vi "Wait For Trigger.vi"(8 "error in":errorcluster, 10 "Cancel":bool, 11 "VISA resource name":refnum<visa-resource-name>) -> (0 "error out":errorcluster, 2 "Trigger Activated":bool, 3 "VISA resource name out":refnum<visa-resource-name>)   [LabVIEW 2020]
uses:
  <vilib>/Instr/_visa.llb/VISA Flush IO Buffer Mask.ctl
panel:
  out "read buffer":string
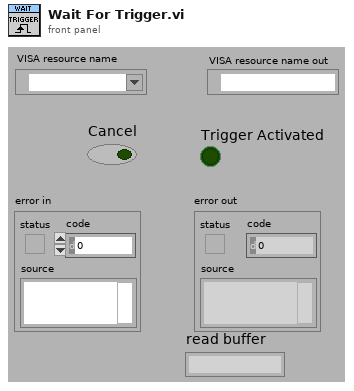
[diagram p1: front panel]
types:
  T1 = typedef "VISA Flush IO Buffer Mask.ctl" = u16
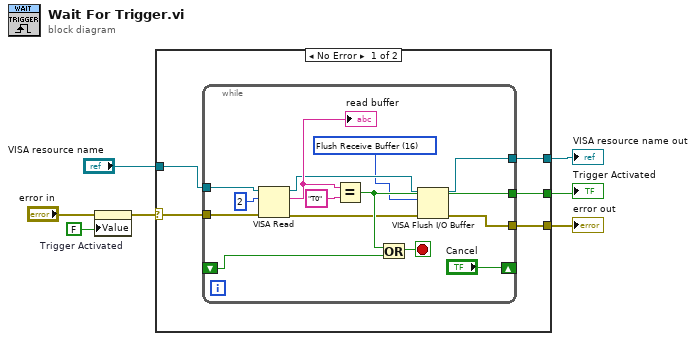
[diagram p0: block diagram]
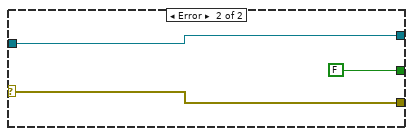
[diagram p2: hidden frame]
diagram:
  n1 = property on="Trigger Activated" class="Bool (strict)"(error in="error in", "Value"=FALSE ("Trigger Activated")) -> (error out=w3:errorcluster)  [unwired: 1 in, 1 out]
  n2 = case shown="No Error" w3 {
    selector: w3 -> [w10 w28]
    tunnel: "VISA resource name" -> [w12 w29]
    tunnel: [w9 w29] -> w6
    tunnel: [w8 w28] -> w5
    tunnel: [w11 FALSE] -> w4
    frame No Error {
      n3 = while {
        tunnel: w12 -> [w26]
        tunnel: w10 -> [w25]
        tunnel: [w20] -> w11
        tunnel: [w18] -> w8
        tunnel: [w16] -> w9
        shift-right: ["Cancel"] -> _
        shift-left: _ -> [w13]
        stop <- w21 stop-if-true
        w15 = T1 16 items=["Flush Receive Buffer"=16, "Write Transmit Buffer to Device"=32, "Flush Receive Buffer (No I/O)"=64, "Flush Transmit Buffer"=128] ("Mask")
        n4 = VISA Read(VISA resource name=w26, byte count=u32 2, error in (no error)=w25) -> (VISA resource name out=w17:refnum<visa-resource-name>, read buffer=w23:string, error out=w19:errorcluster)  [unwired: 1 out]
        "read buffer" <- w23
        n5 = Equal?(x=w23, y="T0") -> (x = y?=w20:bool)
        n6 = Or(x=w20, y=w13) -> (x .or. y?=w21:bool)
        n7 = VISA Flush I/O Buffer(VISA resource name=w17, mask (16)=w15, error in (no error)=w19) -> (VISA resource name out=w16:refnum<visa-resource-name>, error out=w18:errorcluster)
      }
    }
    frame Error {
    }
  }
  "VISA resource name out" <- w6
  "error out" <- w5
  "Trigger Activated" <- w4
